vi "Is Available.vi"(8 "error in (no error)":errorcluster, 11 "LVUnit Test Framework in":refnum<class "LVUnit Test Framework.lvclass">) -> (0 "error out":errorcluster, 2 "Is Available":bool, 3 "LVUnit Test Framework out":refnum<class "LVUnit Test Framework.lvclass">)   [LabVIEW 2017, in "Framework.lvlib" / "LVUnit Test Framework.lvclass"]
doc: "Indicates whether the test framework is currently available. This method must not directly link to the test framework."
uses:
  LVUnit Test Framework.lvclass
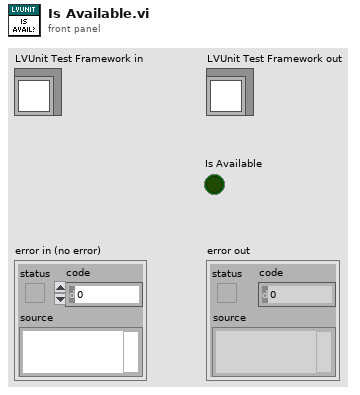
[diagram p1: front panel]
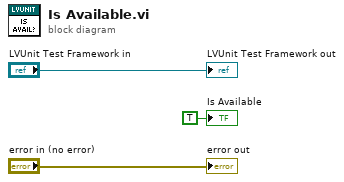
[diagram p0: block diagram]
diagram:
  "error out" <- "error in (no error)"
  "LVUnit Test Framework out" <- "LVUnit Test Framework in"
  "Is Available" <- TRUE ("Is Available")
